vi "Write DragDrop Allow Dropping.vi"(8 "error in (no error)":errorcluster, 10 "AllowDropping":bool, 11 "MulticolumnListbox.lvclass in":refnum<class "MulticolumnListbox.lvclass">) -> (0 "error out":errorcluster, 3 "MulticolumnListbox.lvclass out":refnum<class "MulticolumnListbox.lvclass">)   [LabVIEW 2015, in "MulticolumnListbox.lvclass"]
uses:
  MulticolumnListbox.lvclass
  MulticolumnListbox.lvclass/MulticolumnListbox.ctl
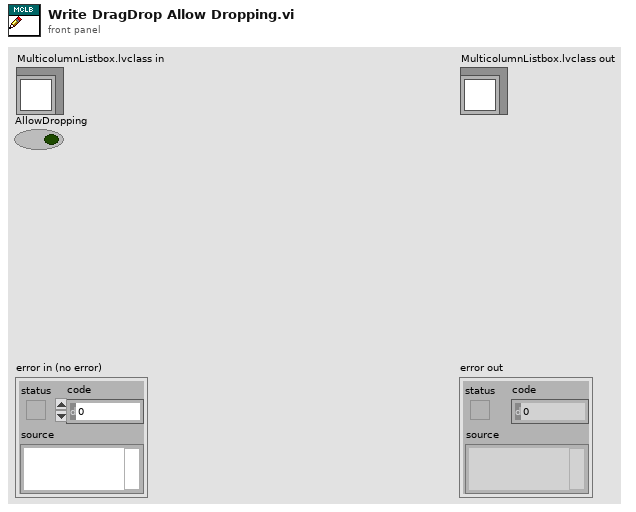
[diagram p1: front panel]
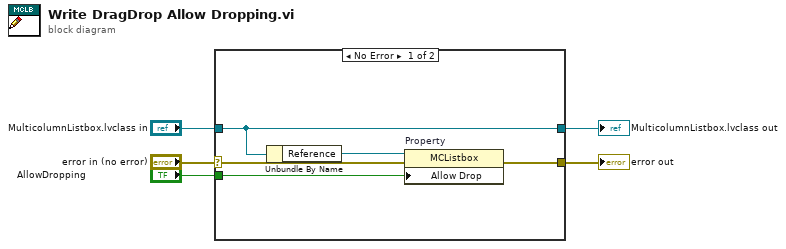
[diagram p0: block diagram]
diagram:
  n1 = case shown="No Error" "error in (no error)" {
    selector: "error in (no error)" -> [w6 w12]
    tunnel: [w10 w12] -> w4
    tunnel: [w8 w11] -> w2
    tunnel: "MulticolumnListbox.lvclass in" -> [w8 w11]
    tunnel: "AllowDropping" -> [w9 _]
    frame No Error {
      n2 = Unbundle By Name(w8) -> ("Reference"=w7:refnum<vi>)
      n3 = property on="Property" class="MCListbox"(reference=w7, error in=w6, "Allow Drop"=w9) -> (error out=w10:errorcluster)  [unwired: 1 out]
    }
    frame Error {
    }
  }
  "error out" <- w4
  "MulticolumnListbox.lvclass out" <- w2
